vi "Sequence Structures.vi"() -> ()   [LabVIEW 2018]
panel:
  out "(C+D)/[2*(C+D)]":dbl
  out "2*(C+D)":dbl
  out "C+D":dbl
  in  "D":dbl
  in  "C":dbl
  out "(A+B)/[2*(A+B)]":dbl
  out "2*(A+B)":dbl
  out "A+B":dbl
  in  "B":dbl
  in  "A":dbl
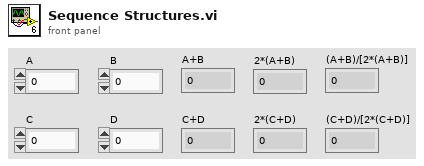
[diagram p1: front panel]
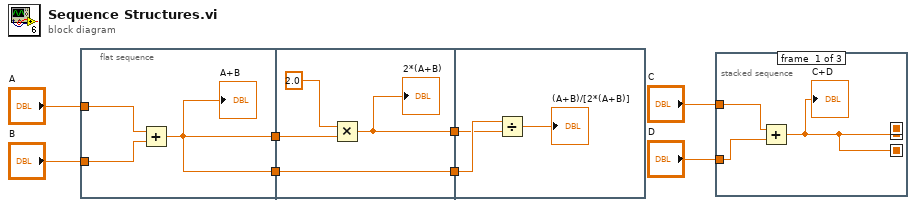
[diagram p0: block diagram]
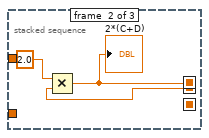
[diagram p2: hidden frame]
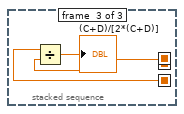
[diagram p3: hidden frame]
diagram:
  n1 = flat-sequence {
    tunnel: "A" -> [w11]
    tunnel: "B" -> [w10]
    tunnel: [w9] -> w6
    tunnel: [w9] -> w5
    tunnel: w6 -> [w14]
    tunnel: w5 -> [w13]
    tunnel: [w13] -> w4
    tunnel: [w12] -> w3
    tunnel: w4 -> [w17]
    tunnel: w3 -> [w16]
    frame #0 {
      n2 = Add(x=w11, y=w10) -> (x+y=w9:dbl)
      "A+B" <- w9
    }
    frame #1 {
      n3 = Multiply(x=2.0, y=w14) -> (x*y=w12:dbl)
      "2*(A+B)" <- w12
    }
    frame #2 {
      n4 = Divide(x=w17, y=w16) -> (x/y=→"(A+B)/[2*(A+B)]":dbl)
    }
  }
  n5 = stacked-sequence {
    seq-local: [w19 _ _] -> [_ w24 _]
    seq-local: [w19 _ _] -> [_ w23 _]
    seq-local: [_ w23 _] -> [_ _ w27]
    seq-local: [_ w22 _] -> [_ _ w26]
    tunnel: "C" -> [w21 _ _]
    tunnel: "D" -> [w20 _ _]
    frame #0 {
      n6 = Add(x=w21, y=w20) -> (x+y=w19:dbl)
      "C+D" <- w19
    }
    frame #1 {
      n7 = Multiply(x=2.0, y=w24) -> (x*y=w22:dbl)
      "2*(C+D)" <- w22
    }
    frame #2 {
      n8 = Divide(x=w27, y=w26) -> (x/y=→"(C+D)/[2*(C+D)]":dbl)
    }
  }
